vi "addToTreeCtl.vi"(4 "AppendToEnd":bool, 6 "ParentTreeTag":string, 7 "glyphArray":string[](array[string]), 8 "error in (no error)":errorcluster, 10 "TreeCtl*":refnum<vi>, 11 "xceDataNode in":refnum<class "xceDataNode.lvclass">) -> (0 "error out":errorcluster, 3 "xceDataNode out":refnum<class "xceDataNode.lvclass">)   [LabVIEW 2013, in "xceDataNode.lvclass"]
doc: "Adds a tree item to a tree control that represents the xceDataNode. Use the glph array input if you wish to have an glyph."
uses:
  xceDataNode.lvclass
  xceTreeObj/xceTreeObj.lvclass
  xceNode/xceNode.lvclass
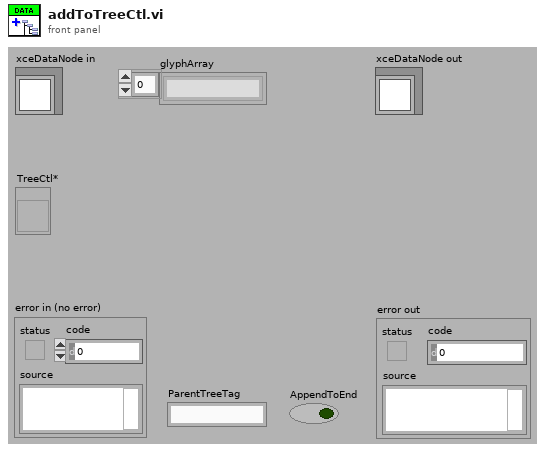
[diagram p1: front panel]
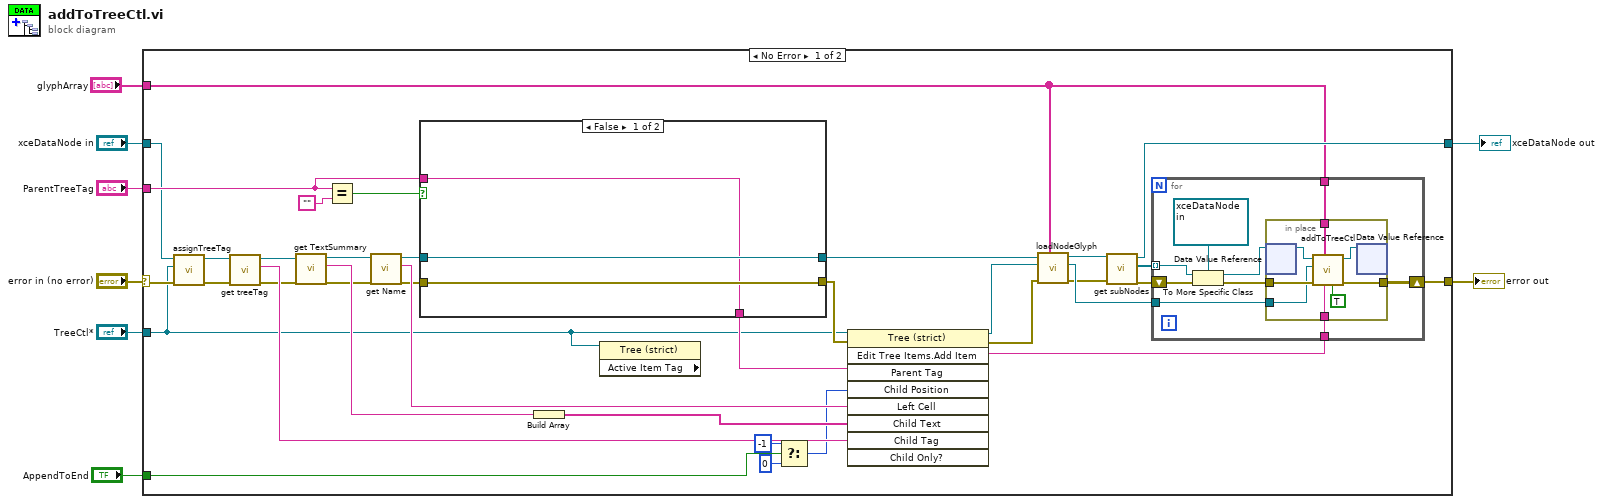
[diagram p0: block diagram]
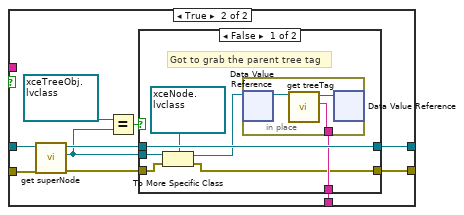
[diagram p2: hidden frame]
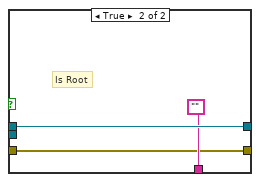
[diagram p3: hidden frame]
diagram:
  n1 = case shown="No Error" "error in (no error)" {
    selector: "error in (no error)" -> [w23 w89]
    tunnel: [w40 w89] -> w5
    tunnel: "xceDataNode in" -> [w24 w88]
    tunnel: "TreeCtl*" -> [w9 _]
    tunnel: "ParentTreeTag" -> [w30 _]
    tunnel: [w22 w88] -> w3
    tunnel: "AppendToEnd" -> [w20 _]
    tunnel: "glyphArray" -> [w10 _]
    frame No Error {
      n2 = call "assignTreeTag.vi"("error in (no error)"=w23, "TreeCtl*"=w9, "xceDataNode in"=w24) -> ("error out"=w26:errorcluster, "xceDataNode out"=w25:refnum<class "xceDataNode.lvclass">)  [unwired: 7 in]
      n3 = call "get treeTag.vi"("error in (no error)"=w26, "xceNode in"=w25) -> ("error out"=w39:errorcluster, "treeTag"=w44:string, "xceNode out"=w36:refnum<class "xceDataNode.lvclass">)  [unwired: 7 in]
      n4 = call-dynamic "get TextSummary.vi"("error in (no error)"=w39, "xceDataNode in"=w36) -> ("error out"=w37:errorcluster, "Text Summary"=w42:string, "xceDataNode out"=w38:refnum<class "xceDataNode.lvclass">)  [unwired: 7 in]
      n5 = Equal?(x=w30, y="") -> (x = y?=w32:bool)
      n6 = call "get Name.vi"("error in (no error)"=w37, "xceDataNode in"=w38) -> ("error out"=w34:errorcluster, "Name"=w43:string, "xceDataNode out"=w33:refnum<class "xceDataNode.lvclass">)  [unwired: 7 in]
      n7 = case shown="False" w32 {
        tunnel: w34 -> [w46 w57]
        tunnel: w33 -> [w47 w56]
        tunnel: [w47 w52] -> w15
        tunnel: [w45 w50] -> w31
        tunnel: [w46 w48] -> w28
        tunnel: w30 -> [w45 _]
        frame False {
        }
        frame True {
          n8 = call "get superNode.vi"("error in (no error)"=w57, "xceNode in"=w56) -> ("error out"=w49:errorcluster, "superNode*"=w51:refnum<data-value>, "xceNode out"=w53:refnum<class "xceDataNode.lvclass">)  [unwired: 7 in]
          n9 = Equal?(x=refnum<data-value> refnum, y=w51) -> (x = y?=w54:bool)
          n10 = case shown="False" w54 {
            tunnel: w53 -> [w64 w70]
            tunnel: [w64 w70] -> w52
            tunnel: w51 -> [w63 _]
            tunnel: [w60 ""] -> w50
            tunnel: w49 -> [w59 w68]
            tunnel: [w58 w68] -> w48
            frame False {
              # "Got to grab the parent tree tag"
              n11 = To More Specific Class(target class=refnum<data-value> refnum ("data value reference"), reference=w63, error in=w59) -> (specific class reference=w61:refnum<data-value>, error out=w58:errorcluster)
              n12 = in-place {
                in-place-border: [w65] -> w60
                n13 = in-place-dvr #1(w61) -> (w67:refnum<class "xceNode.lvclass">)  [unwired: 1 out]
                n14 = call "get treeTag.vi"("xceNode in"=w67) -> ("treeTag"=w65:string, "xceNode out"=w66:refnum<class "xceNode.lvclass">)  [unwired: 8 in, 1 out]
                n15 = in-place-dvr #1(w66) -> ()  [unwired: 2 out]
              }
            }
            frame True {
              # "Is Root"
            }
          }
        }
      }
      n16 = Build Array(w42) -> (w41:string[])
      n17 = property class="Tree (strict)" props=["Active Item Tag"](reference=w9) -> ()  [unwired: 1 in, 3 out]
      n18 = Select(t=-1, s=w20, f=0 ("Child Position")) -> (s? t:f=w17:i32)
      n19 = invoke class="Tree (strict)" method="Edit Tree Items.Add Item"(reference=w9, error in=w28, "Parent Tag"=w31, "Child Position"=w17, "Left Cell"=w43, "Child Text"=w41, "Child Tag"=w44) -> (reference out=w14:refnum<vi>, error out=w12:errorcluster, "Edit Tree Items:Add Item"=w21:string)  [unwired: 2 in, 6 out]
      n20 = call "loadNodeGlyph.vi"("glyphArray"=w10, "error in (no error)"=w12, "TreeCtl* in"=w14, "xceDataNode in"=w15) -> ("error out"=w11:errorcluster, "TreeCtl* out"=w13:refnum<vi>, "xceDataNode out"=w16:refnum<class "xceDataNode.lvclass">)  [unwired: 5 in]
      n21 = call "get subNodes.vi"("error in (no error)"=w11, "xceNode in"=w16) -> ("error out"=w27:errorcluster, "subNodes[]*"=w29:refnum<data-value>[], "xceNode out"=w22:refnum<class "xceDataNode.lvclass">)  [unwired: 7 in]
      n22 = for {
        tunnel: w29 -> [w77] mode=indexing
        shift-right: [w74] -> w40
        shift-left: w27 -> [w79]
        tunnel: w13 -> [w73]
        tunnel: w21 -> [w72]
        tunnel: w10 -> [w71]
        n23 = To More Specific Class(target class=refnum<data-value> refnum ("data value reference"), reference=w77, error in=w79) -> (specific class reference=w75:refnum<data-value>, error out=w78:errorcluster)
        n24 = in-place {
          in-place-border: w78 -> [w87]
          in-place-border: [w86] -> w74
          in-place-border: w73 -> [w83]
          in-place-border: w72 -> [w82]
          in-place-border: w71 -> [w81]
          n25 = in-place-dvr #2(w75) -> (w85:refnum<class "xceDataNode.lvclass">)  [unwired: 1 out]
          n26 = call "addToTreeCtl.vi"("AppendToEnd"=TRUE, "ParentTreeTag"=w82, "glyphArray"=w81, "error in (no error)"=w87, "TreeCtl*"=w83, "xceDataNode in"=w85) -> ("error out"=w86:errorcluster, "xceDataNode out"=w84:refnum<class "xceDataNode.lvclass">)  [unwired: 4 in]
          n27 = in-place-dvr #2(w84) -> ()  [unwired: 2 out]
        }
      }
    }
    frame Error {
    }
  }
  "xceDataNode out" <- w3
  "error out" <- w5
